vi "Append Report Text (str wrap).vi"(0 "report in":refnum<class "NI_report.lvclass"> caption="报表输入", 1 "MS Office parameters":T1 caption="MS Office参数", 2 "format string (%.3f)":string="%.3f" caption="格式字符串(%.3f)", 7 "text":string caption="文本", 9 "append on new line? (F)":bool caption="添加至新行？(F)", 11 "error in (no error)":errorcluster caption="错误输入（无错误）") -> (4 "report out":refnum<class "NI_report.lvclass"> caption="报表输出", 8 "start out (Word)":i32 caption="开始输出(Word)", 10 "end out (Word)":i32 caption="结束输出(Word)", 15 "error out":errorcluster caption="错误输出")   [LabVIEW 2018]
doc: "添加文本至所选报表。 通过连线数据至<B>文本</B>输入端可确定要使用的多态实例，也可手动选择实例。"
uses:
  <vilib>/Utility/NIReport.llb/NI_report.lvclass
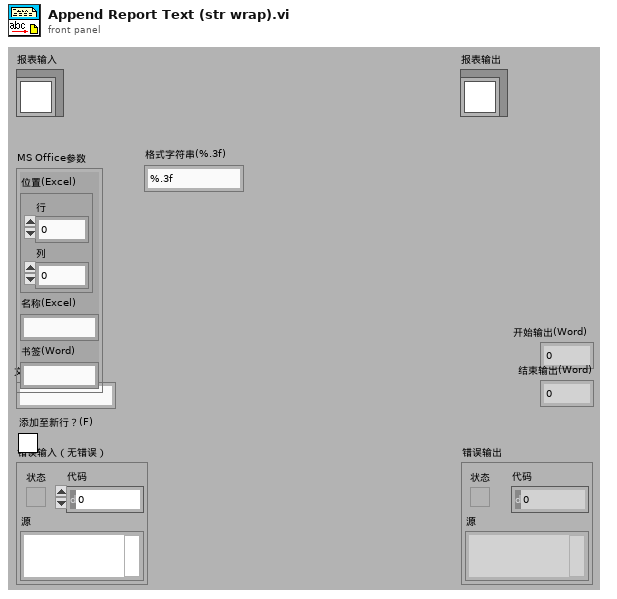
[diagram p1: front panel]
types:
  T1 = cluster{"position (excel)":cluster{"row":i32, "column":i32}, "name (excel)":string, "bookmark (word)":string}
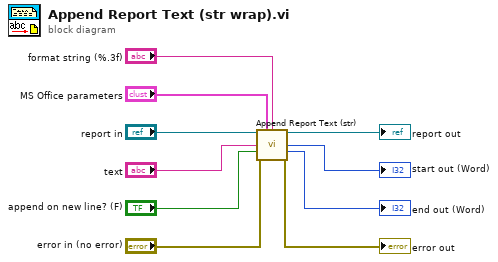
[diagram p0: block diagram]
diagram:
  n1 = call-dynamic "Append Report Text (str).vi"("report in"="report in", "MS Office parameters"="MS Office parameters", "format string (%.3f)"="format string (%.3f)", "text"="text", "append on new line? (F)"="append on new line? (F)", "error in (no error)"="error in (no error)") -> ("report out"=→"report out":refnum<class "NI_report.lvclass">, "start out (Word)"=→"start out (Word)":i32, "end out (Word)"=→"end out (Word)":i32, "error out"=→"error out":errorcluster)  [unwired: 6 out]
